vi "open in notepad.vi"(7 "wait until completion? (T)":bool, 8 "error in (no error)":errorcluster, 11 "Path":path) -> (0 "error out":errorcluster)   [LabVIEW 2014]
doc: "This subVI opens a txt file in notepad. \nDefault Path is the relative path of file to this VI which is used for development mode. In Run Time mode (running the executable version), Run Time Path is used to open the file."
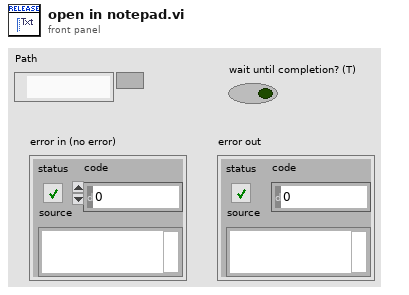
[diagram p1: front panel]
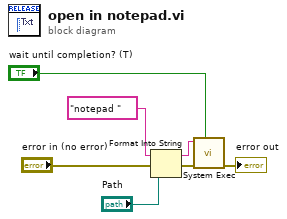
[diagram p0: block diagram]
diagram:
  n1 = Format Into String(initial string="notepad ", error in="error in (no error)", "Path") -> (resulting string=w4:string, error out=w5:errorcluster)  [unwired: 1 in]
  n2 = call <vilib>:"System Exec.vi"("wait until completion? (T)"="wait until completion? (T)", "error in (no error)"=w5, "command line"=w4) -> ("error out"=→"error out":errorcluster)  [unwired: 5 in, 3 out]
